vi "Prepare Bus Monitor Interface.vi"(9 "Datum Name":string, 11 "ListboxBusMonitor":refnum<class "ListboxBusMonitor.lvclass">) -> (2 "Valid Transport":refnum<class "ITransport.lvclass">, 3 "SubscriptionPolicy":refnum<class "ISubscriptionPolicy.lvclass">)   [LabVIEW 2017, in "ListboxBusMonitor.lvlib" / "ListboxBusMonitor.lvclass"]
uses:
  ListboxBusMonitor.lvclass
  gpm_packages/@cs/transport/Source/ITransport/ITransport.lvclass
  gpm_packages/@cs/mva-core/Source/IMediator/ISubscriptionPolicy/ISubscriptionPolicy.lvclass
  ListboxBusMonitor.lvclass/ListboxBusMonitor.ctl
  ListboxBusMonitorPanel Messages/Update Monitored Datum Msg/Update Monitored Datum Msg.lvclass
  C:/Git/mva-framework/gpm_packages/@cs/transport/Source/Concrete/ActorMessageTransport/Notification Msg/Notification Msg.lvclass
  gpm_packages/@cs/mva-core/Source/SubscriptionPolicy/BasicSubscription/BasicSubscription.lvclass/BasicSubscription.ctl
  gpm_packages/@cs/transport/Source/Concrete/ActorMessageTransport/ActorMessageTransport.lvclass/ActorMessageTransport.ctl
  <vilib>/ActorFramework/Message Enqueuer/Equals Not A Refnum.vi
  gpm_packages/@cs/mva-core/Source/SubscriptionPolicy/BasicSubscription/BasicSubscription.lvclass
  C:/Git/mva-framework/gpm_packages/@cs/mva-core/Source/IMediator/ISubscriptionPolicy/ISubscriptionPolicy.lvclass
  gpm_packages/@cs/transport/Source/Concrete/ActorMessageTransport/ActorMessageTransport.lvclass
  C:/Git/mva-framework/gpm_packages/@cs/transport/Source/ITransport/ITransport.lvclass
  <vilib>/Utility/error.llb/Error Cluster From Error Code.vi
  <vilib>/ActorFramework/Message Enqueuer/Message Enqueuer.lvclass
  gpm_packages/@cs/transport/Source/Concrete/ActorMessageTransport/Notification Msg/Notification Msg.lvclass
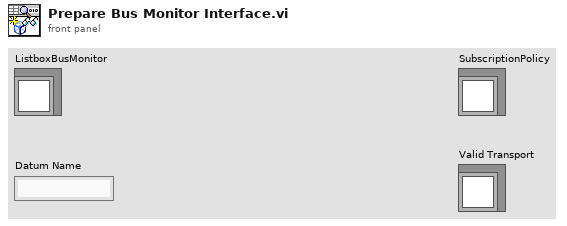
[diagram p1: front panel]
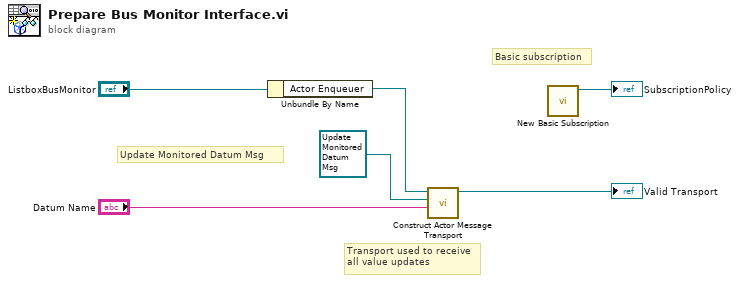
[diagram p0: block diagram]
diagram:
  # "Basic subscription"
  # "Transport used to receive\nall value updates"
  # "Update Monitored Datum Msg"
  n1 = Unbundle By Name("ListboxBusMonitor") -> ("Actor Enqueuer"=w1:refnum<class "Message Enqueuer.lvclass">)
  n2 = call "Construct Actor Message Transport.vi"("Datum Name"="Datum Name", "Notification Msg"=refnum<class "Update Monitored Datum Msg.lvclass"> refnum ("ListboxBusMonitor.lvlib:Update Monitored Datum Msg.lvclass"), "Message Enqueuer in"=w1) -> ("ActorMessageTransport"=→"Valid Transport":refnum<class "ActorMessageTransport.lvclass">)  [unwired: 7 in, 1 out]
  n3 = call "New Basic Subscription.vi"() -> ("BasicSubscription Out"=→"SubscriptionPolicy":refnum<class "BasicSubscription.lvclass">)  [unwired: 11 in]
